vi "Add Resistive card.vi"(8 "error in (no error)":errorcluster, 11 "Node Ptr":u64 format="%.0x") -> (0 "error out":errorcluster)   [LabVIEW 2014, in "SLSC configuration System Explorer.lvlib"]
uses:
  SLSC configuration System Explorer.lvlib
  <vilib>/NI Veristand/Custom Device API/Custom Device API.lvlib
  Shared/Constants.vi
  Shared/SLSC configuration Shared.lvlib
  <vilib>/NI Veristand/Custom Device API/Set Item Property (Variant).vi
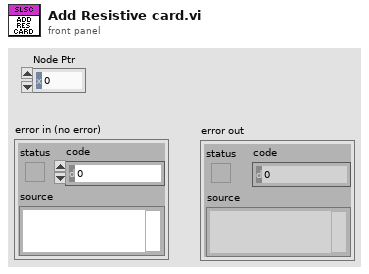
[diagram p1: front panel]
types:
  T1 = typedef "SLSC configuration Shared.lvlib/Slot #.ctl" = u8
  T2 = typedef "Custom Device API.lvlib/Custom Device Item Ref.ctl" = u64
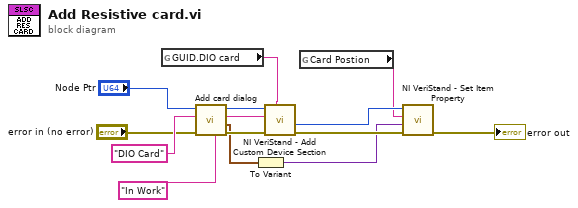
[diagram p0: block diagram]
diagram:
  n1 = global read "Constants.vi" "GUID.DIO card"() -> (w13:string)
  n2 = call "Add card dialog.vi"("Cancelled?"="In Work" ("Section Name"), "error in (no error)"="error in (no error)", "Card Type in"="DIO Card" ("Section Name"), "Node Ptr"="Node Ptr") -> ("error out"=w9:errorcluster, "Card Position out"=w4:cluster{"Rack #":u8, "Slot #":T1}, "Name out"=w8:string, "Node Ptr out"=w7:u64)  [unwired: 4 in]
  n3 = To Variant(anything=w4) -> (Variant=w3:variant)
  n4 = call <vilib>:"NI VeriStand - Add Custom Device Section.vi"("GUID (Default Section)"=w13, "error in (no error)"=w9, "Section Name"=w8, "Parent Ref in"=w7) -> ("error out"=w14:errorcluster, "Section Ptr"=w5:T2)  [unwired: 4 in, 2 out]
  n5 = global read "Constants.vi" "Card Postion"() -> (w2:string)
  n6 = call-poly <vilib>:"NI VeriStand - Set Item Property.vi"("error in (no error)"=w14, "Value"=w3, "Property Name"=w2, "Item Ref in"=w5) -> ("error out"=→"error out":errorcluster)  [unwired: 5 in, 2 out]
